vi "Write Col Data.vi"(6 "Insert If Not Exist(T)":bool=TRUE, 7 "Section Name":string, 8 "error in (no error)":errorcluster, 9 "Column Data":string[](array[string]), 10 "Col Header Name":string, 11 "Config Data":T1(array[cluster])) -> (0 "error out":errorcluster, 3 "Config Data dup":T1(array[cluster]), 4 "Find?":bool)   [LabVIEW 2020, in "GUCalibration2.lvlib"]
uses:
  GUCalibration2.lvlib
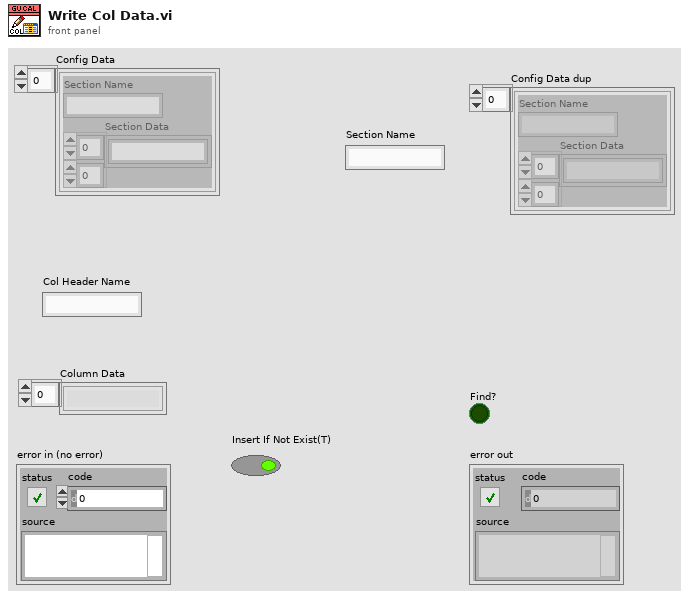
[diagram p1: front panel]
types:
  T1 = cluster{"Section Name":string, "Section Data":string[][]}[]
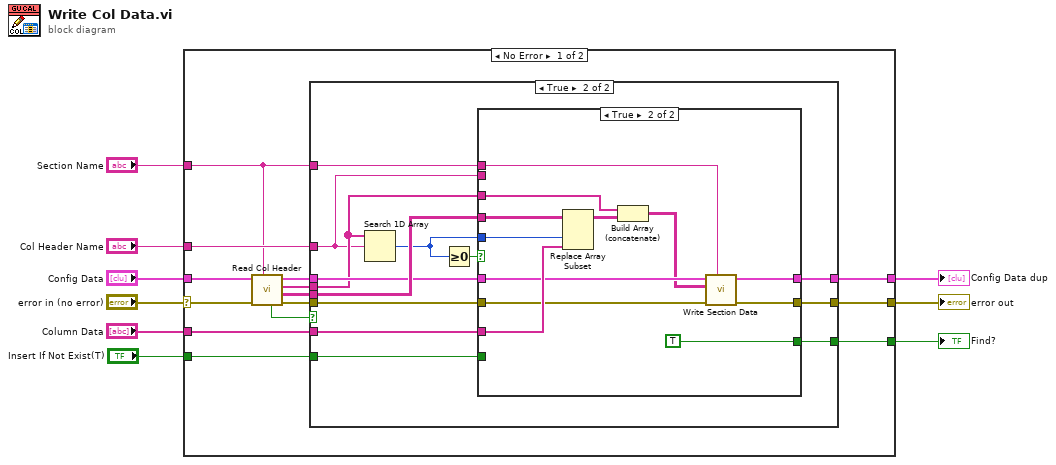
[diagram p0: block diagram]
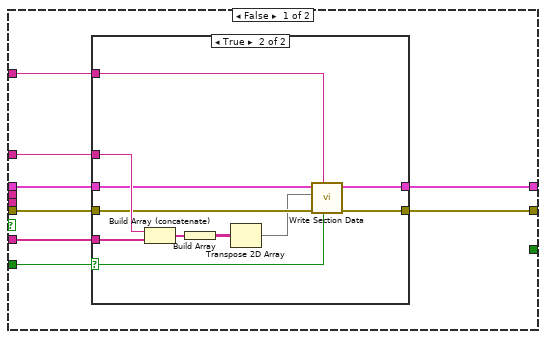
[diagram p2: hidden frame]
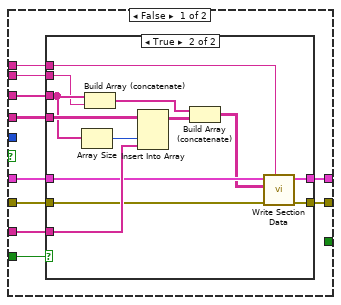
[diagram p4: hidden frame]
diagram:
  n1 = case shown="No Error" "error in (no error)" {
    selector: "error in (no error)" -> [w22 w96]
    tunnel: "Section Name" -> [w16 _]
    tunnel: "Config Data" -> [w23 w95]
    tunnel: [w15 w96] -> w6
    tunnel: [w14 w95] -> w1
    tunnel: "Col Header Name" -> [w21 _]
    tunnel: "Column Data" -> [w19 _]
    tunnel: "Insert If Not Exist(T)" -> [w11 _]
    tunnel: [w10 _] -> w2
    frame No Error {
      n2 = call "Read Col Header.vi"("Section Name"=w16, "error in (no error)"=w22, "Config Data"=w23) -> ("error out"=w17:errorcluster, "Data"=w20:string[][], "Column Header"=w13:string[], "Config Data dup"=w18:T1, "Section Find?"=w12:bool)  [unwired: 4 in]
      n3 = case shown="True" w12 {
        tunnel: w21 -> [w31 w47]
        tunnel: w20 -> [_ w57]
        tunnel: w19 -> [w30 w55]
        tunnel: w18 -> [w24 w54]
        tunnel: w17 -> [w28 w53]
        tunnel: w16 -> [w25 w52]
        tunnel: [w27 w51] -> w15
        tunnel: [w26 w50] -> w14
        tunnel: w13 -> [_ w49]
        tunnel: w11 -> [w29 w46]
        tunnel: [_ w45] -> w10
        frame False {
          n4 = case shown="True" w29 {
            selector: w29 -> [_ w34]
            tunnel: w31 -> [_ w44]
            tunnel: w30 -> [_ w43]
            tunnel: w28 -> [w32 w40]
            tunnel: [w32 w39] -> w27
            tunnel: [w33 w38] -> w26
            tunnel: w25 -> [_ w37]
            tunnel: w24 -> [w33 w35]
            frame False {
            }
            frame True {
              n5 = Build Array (concatenate)(w44, w43) -> (w42:string[])
              n6 = Build Array(w42) -> (w41:string[][])
              n7 = Transpose 2D Array(2D array=w41) -> (transposed array=w36:string[][])
              n8 = call "Write Section Data.vi"("Insert If Not Exist(T)"=w34, "Section Name"=w37, "error in (no error)"=w40, "Section Data"=w36, "Config Data"=w35) -> ("error out"=w39:errorcluster, "Config Data out"=w38:T1)  [unwired: 5 in]
            }
          }
        }
        frame True {
          n9 = Search 1D Array(1D array=w49, element=w47) -> (index of element=w56:i32)  [unwired: 1 in]
          n10 = Greater Or Equal To 0?(x=w56) -> (x >= 0?=w48:bool)
          n11 = case shown="True" w48 {
            tunnel: w57 -> [w67 w94]
            tunnel: w56 -> [_ w83]
            tunnel: w55 -> [w66 w93]
            tunnel: w54 -> [w63 w91]
            tunnel: w53 -> [w64 w92]
            tunnel: w52 -> [w59 w90]
            tunnel: [w62 w89] -> w51
            tunnel: [w61 w88] -> w50
            tunnel: w49 -> [w65 w87]
            tunnel: w47 -> [w60 _]
            tunnel: w46 -> [w58 _]
            tunnel: [_ TRUE] -> w45
            frame False {
              n12 = case shown="True" w58 {
                tunnel: w67 -> [_ w82]
                tunnel: w66 -> [_ w81]
                tunnel: w65 -> [_ w80]
                tunnel: w64 -> [w69 w76]
                tunnel: w63 -> [w68 w75]
                tunnel: [w69 w74] -> w62
                tunnel: [w68 w73] -> w61
                tunnel: w60 -> [_ w72]
                tunnel: w59 -> [_ w70]
                frame False {
                }
                frame True {
                  n13 = Array Size(array=w80) -> (size(s)=w79:i32)
                  n14 = Build Array (concatenate)(w80, w72) -> (w78:string[])
                  n15 = Insert Into Array(array=w82, index (col)=w79, new element=w81) -> (w77:string[][])  [unwired: 1 in]
                  n16 = Build Array (concatenate)(w78, w77) -> (w71:string[][])
                  n17 = call "Write Section Data.vi"("Section Name"=w70, "error in (no error)"=w76, "Section Data"=w71, "Config Data"=w75) -> ("error out"=w74:errorcluster, "Config Data out"=w73:T1)  [unwired: 6 in]
                }
              }
            }
            frame True {
              n18 = Replace Array Subset(array=w94, new element=w93, index (col)=w83) -> (w86:string[][])  [unwired: 1 in]
              n19 = Build Array (concatenate)(w87, w86) -> (w85:string[][])
              n20 = call "Write Section Data.vi"("Section Name"=w90, "error in (no error)"=w92, "Section Data"=w85, "Config Data"=w91) -> ("error out"=w89:errorcluster, "Config Data out"=w88:T1)  [unwired: 6 in]
            }
          }
        }
      }
    }
    frame Error {
    }
  }
  "error out" <- w6
  "Config Data dup" <- w1
  "Find?" <- w2
